vi "Find Plugin.vi"(8 "error in":errorcluster, 10 "name":string, 11 "plugins":T1[](array[typedef])) -> (0 "error out":errorcluster, 1 "found?":bool, 2 "index":i32, 3 "plugins out":T1[](array[typedef]))   [LabVIEW 2020, in "DSF Configuration API.lvlib"]
uses:
  DSF Configuration API.lvlib
  68c4a88d-ce08-4724-b515-f9b610a0f92e.vi
  Includes/DSF Core.lvlibp/Typedefs/DSF Timing Info.ctl
  Includes/DSF Core.lvlibp
  Includes/DSF Core.lvlibp/Typedefs/Core Plugin Configuration.ctl
  Includes/DSF Core.lvlibp/Classes/Configuration/Core/Plugin/Plugin Configuration.lvclass
  Includes/DSF Core.lvlibp/Typedefs/DSF Settings Info.ctl
  Includes/DSF Core.lvlibp/Typedefs/Core Thread Configuration.ctl
  Includes/DSF Core.lvlibp/Classes/Configuration/Core/Thread/Thread Configuration.lvclass
  Includes/DSF Core.lvlibp/Typedefs/DSF Direction.ctl
  Includes/DSF Core.lvlibp/Typedefs/DSF Timeout Behavior.ctl
  Includes/DSF Core.lvlibp/Typedefs/Core Group Configuration.ctl
  Includes/DSF Core.lvlibp/Classes/Configuration/Core/Group/Group Configuration.lvclass
  Includes/DSF Core.lvlibp/Typedefs/Core Transfer Configuration.ctl
  Includes/DSF Core.lvlibp/Classes/Configuration/Core/Transfer/Transfer Configuration.lvclass
  Includes/DSF Core.lvlibp/Typedefs/DSF Data Type.ctl
  Includes/DSF Core.lvlibp/Typedefs/Core Channel Configuration.ctl
  Includes/DSF Core.lvlibp/Classes/Configuration/Core/Channel/Channel Configuration.lvclass
  Includes/DSF Core.lvlibp/Typedefs/DSF Engine Channel Configuration.ctl
  Includes/DSF Core.lvlibp/Typedefs/DSF Engine Transfer Configuration.ctl
  Includes/DSF Core.lvlibp/Typedefs/DSF Engine Transfer Group Configuration.ctl
  Includes/DSF Core.lvlibp/Typedefs/DSF Engine Plugin Thread Configuration.ctl
  Includes/DSF Core.lvlibp/Typedefs/DSF Engine Plugin Configuration.ctl
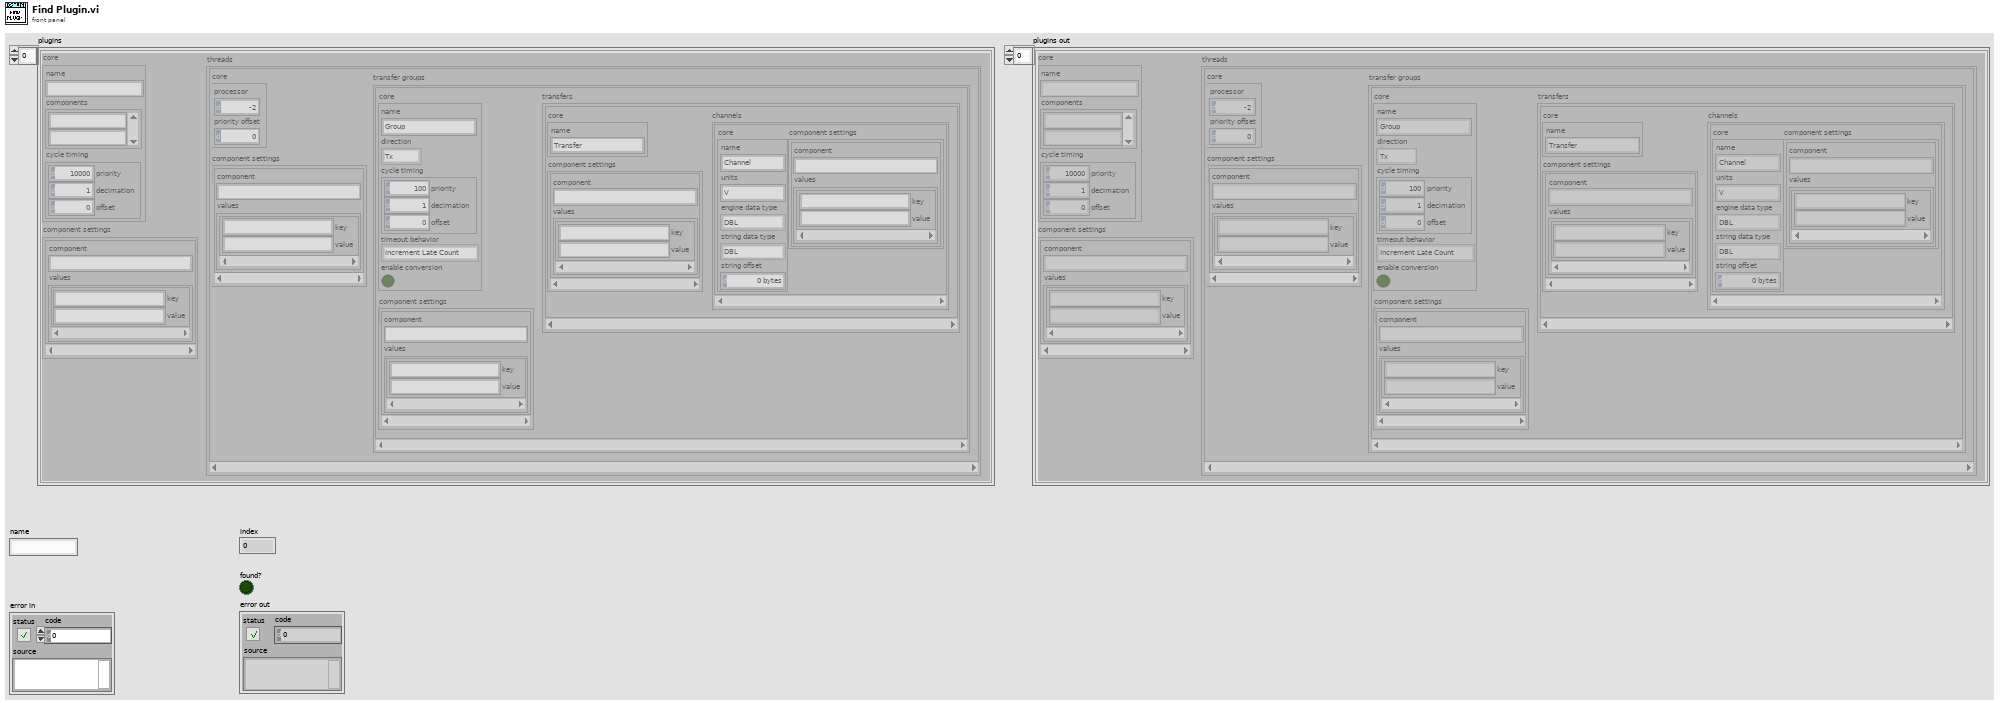
[diagram p1: front panel]
types:
  T1 = typedef "DSF Core.lvlibp/DSF Engine Plugin Configuration.ctl" = cluster{"core":T2, "component settings":T4[], "threads":T5[]}
  T2 = typedef "DSF Core.lvlibp/Plugin Configuration.lvclass/Core Plugin Configuration.ctl" = cluster{"name":string, "components":string[], "cycle timing":T3}
  T3 = typedef "DSF Core.lvlibp/DSF Timing Info.ctl" = cluster{"priority":u64, "decimation":u64, "offset":u64}
  T4 = typedef "DSF Core.lvlibp/DSF Settings Info.ctl" = cluster{"component":string, "values":cluster{"key":string, "value":string}[]}
  T5 = typedef "DSF Core.lvlibp/DSF Engine Plugin Thread Configuration.ctl" = cluster{"core":T6, "component settings":T4[], "transfer groups":T7[]}
  T6 = typedef "DSF Core.lvlibp/Thread Configuration.lvclass/Core Thread Configuration.ctl" = cluster{"processor":i32, "priority offset":i16}
  T7 = typedef "DSF Core.lvlibp/DSF Engine Transfer Group Configuration.ctl" = cluster{"core":T8, "component settings":T4[], "transfers":T11[]}
  T8 = typedef "DSF Core.lvlibp/Group Configuration.lvclass/Core Group Configuration.ctl" = cluster{"name":string, "direction":T9, "cycle timing":T3, "timeout behavior":T10, "enable conversion":bool}
  T9 = typedef "DSF Core.lvlibp/DSF Direction.ctl" = enum8{"Tx", "Rx"}
  T10 = typedef "DSF Core.lvlibp/DSF Timeout Behavior.ctl" = enum8{"Increment Late Count", "Throw Error"}
  T11 = typedef "DSF Core.lvlibp/DSF Engine Transfer Configuration.ctl" = cluster{"core":T12, "component settings":T4[], "channels":T13[]}
  T12 = typedef "DSF Core.lvlibp/Transfer Configuration.lvclass/Core Transfer Configuration.ctl" = cluster{"name":string}
  T13 = typedef "DSF Core.lvlibp/DSF Engine Channel Configuration.ctl" = cluster{"core":T14, "component settings":T4[]}
  T14 = typedef "DSF Core.lvlibp/Channel Configuration.lvclass/Core Channel Configuration.ctl" = cluster{"name":string, "units":string, "engine data type":T15, "string data type":T15, "string offset":u64}
  T15 = typedef "DSF Core.lvlibp/DSF Data Type.ctl" = enum8{"Bool", "SGL", "DBL", "I8", "I16", "I32", "I64", "U8", "U16", "U32", "U64"}
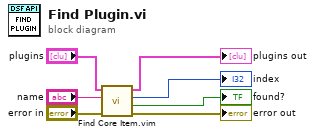
[diagram p0: block diagram]
diagram:
  n1 = call "Find Core Item.vim"("error in"="error in", "item name"="name", "item array"="plugins") -> ("error out"=→"error out":errorcluster, "found?"=→"found?":bool, "index"=→"index":i32, "item array out"=→"plugins out":T1[])  [unwired: 5 in]
